vi "onSuiteSlippage.vi"(7 "DestroySuite in":refnum<class "DestroySuite.lvclass">, 10 "Properties.Suite":refnum<class "Properties.Suite.lvclass">) -> (0 "error out":errorcluster, 2 "Properties.Suite out":refnum<class "Properties.Suite.lvclass">)   [LabVIEW 2021, in "Bananas.lvlib" / "DestroySuite.lvclass"]
uses:
  DestroySuite.lvclass
  <vilib>/addons/_JKI Toolkits/Caraya/classes/Properties.Suite/Properties.Suite.lvclass
  C:/Program Files (x86)/National Instruments/LabVIEW 2021/vi.lib/addons/_JKI Toolkits/Caraya/classes/Properties/Properties.lvclass
  DestroySuite.lvclass/DestroySuite.ctl
  <vilib>/addons/_JKI Toolkits/Caraya/classes/Properties/Properties.lvclass
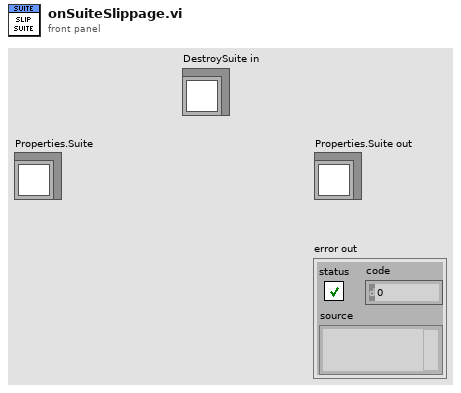
[diagram p1: front panel]
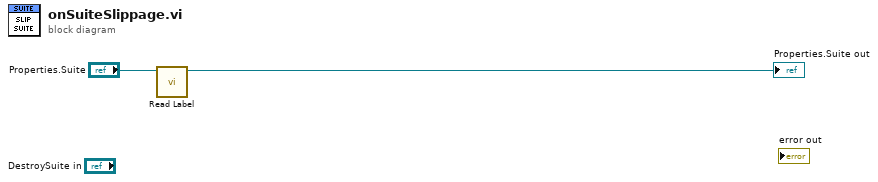
[diagram p0: block diagram]
diagram:
  n1 = call <vilib>:"Read Label.vi"("Properties in"="Properties.Suite") -> ("Properties out"=→"Properties.Suite out":refnum<class "Properties.Suite.lvclass">)  [unwired: 9 in, 1 out]
